vi "InitiateGeneration.vi"(8 "error in (no error)":errorcluster, 11 "DaqMx_Single in":refnum<class "DaqMx_Single.lvclass">) -> (0 "error out":errorcluster, 3 "DaqMx_Single out":refnum<class "DaqMx_Single.lvclass">)   [LabVIEW 2018, in "FgenPlugins.lvlib" / "DaqMx_Single.lvclass"]
uses:
  DaqMx_Single.lvclass
  Private/Run.vi
  <vilib>/Utility/error.llb/Error Cluster From Error Code.vi
  <vilib>/ErrorRing/Error Ring.xnode
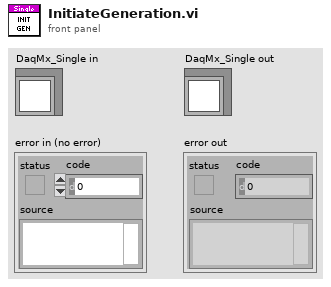
[diagram p1: front panel]
types:
  T1 = enum32{"Bad", "Idle", "Run top level", "Running"}
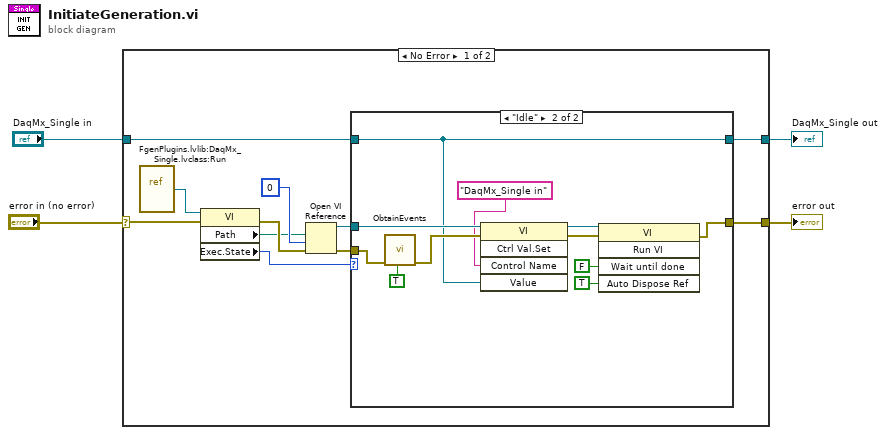
[diagram p0: block diagram]
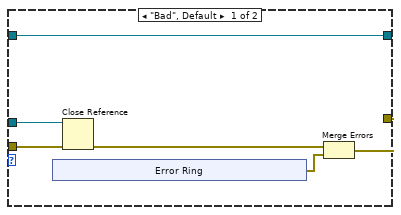
[diagram p2: hidden frame]
diagram:
  n1 = case shown="No Error" "error in (no error)" {
    selector: "error in (no error)" -> [w7 w38]
    tunnel: [w8 w38] -> w3
    tunnel: [w5 w37] -> w1
    tunnel: "DaqMx_Single in" -> [w6 w37]
    frame No Error {
      n2 = vi-ref "FgenPlugins.lvlib:DaqMx_Single.lvclass:Run.vi"() -> (w12:refnum<vi>)
      n3 = property class="VI"(reference=w12, error in=w7) -> (error out=w14:errorcluster, "Path"=w13:path, "Exec.State"=w11:T1)  [unwired: 1 out]
      n4 = Open VI Reference(vi path=w13, options=0, error in (no error)=w14) -> (vi reference=w10:refnum<vi>, error out=w9:errorcluster)  [unwired: 3 in]
      n5 = case shown="\"Idle\"" w11 {
        tunnel: w10 -> [w21 w34]
        tunnel: w9 -> [w20 w36]
        tunnel: [w17 w26] -> w8
        tunnel: w6 -> [w16 w27]
        tunnel: [w16 w27] -> w5
        frame "Bad", Default {
          n6 = xnode "Error Ring"() -> ("error out"=w18:errorcluster)
          n7 = Close Reference(reference=w21, error in (no error)=w20) -> (error out=w19:errorcluster)
          n8 = Merge Errors(w19, w18) -> (w17:errorcluster)
        }
        frame "Idle" {
          n9 = call "ObtainEvents.vi"("Set? (f)"=TRUE, "error in (no error)"=w36) -> ("error out"=w33:errorcluster)  [unwired: 8 in, 1 out]
          n10 = invoke class="VI" method="Ctrl Val.Set"(reference=w34, error in=w33, "Control Name"="DaqMx_Single in", "Value"=w27) -> (reference out=w29:refnum<vi>, error out=w28:errorcluster)  [unwired: 1 in, 3 out]
          n11 = invoke class="VI" method="Run VI"(reference=w29, error in=w28, "Wait until done"=FALSE ("Wait Until Done"), "Auto Dispose Ref"=TRUE ("Auto Dispose Reference")) -> (error out=w26:errorcluster)  [unwired: 1 in, 4 out]
        }
      }
    }
    frame Error {
    }
  }
  "error out" <- w3
  "DaqMx_Single out" <- w1
